vi "Engine_Build.vi"(8 "ErrIn":errorcluster, 9 "Programmatic?":bool, 10 "New item":T1, 11 "IB_MSI.lvclass":refnum<class "IB_MSI.lvclass">) -> (0 "ErrOut":errorcluster, 1 "warning":string, 2 "Canceled?":bool)   [LabVIEW 2020, in "IB_MSI.lvclass"]
uses:
  <vilib>/AppBuilder/IB_Classes/MSI/IB_MSI.lvclass
  AppLibs/distkit/MDF/NI_MDF.lvlib
  <resource>/Framework/Providers/Builds/Installer/CDK_GLOBAL_STRINGS.vi
  AppLibs/distkit/MDF/NIMdf.llb/MDFMIResourceStringID.ctl
  <vilib>/AppBuilder/IB_Classes/Installer/Installer.lvclass
  AppLibs/distkit/MDF/NIMdf.llb/MDFCommonOptions.ctl
  e:/builds/penguin/labview/branches/2020/dev/dist/vi.lib/AppBuilder/IB_Classes/Installer/Installer.lvclass
  e:/builds/penguin/labview/branches/2020/dev/dist/vi.lib/AppBuilder/IB_Classes/MSI/IB_MSI.lvclass
  <resource>/Framework/Providers/API/mxLvBuildNewItem.ctl
panel:
  out "#Vol":u32
  out "VolumeLabel":string
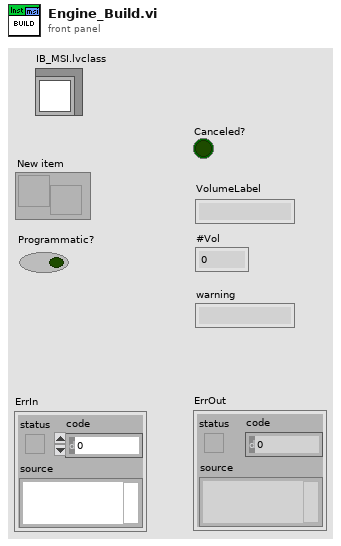
[diagram p1: front panel]
types:
  T1 = typedef "mxLvBuildNewItem.ctl" = refnum<user-event>
  T2 = cluster{"last known path":path, "Index":i32, "DistTitle":string}[]
  T3 = typedef "NI_MDF.lvlib/MDFMIResourceStringID.ctl" = i32
  T4 = typedef "IB_Installer.ctl" = cluster{"Destination":refnum<class "IB_Destination.lvclass">[], "Source":refnum<class "IB_Source.lvclass">[], "buildObject":T5, "defaultDir":string, "platform":string, "author":string, "productName":string, "buildSpecName":string, "hide":bool, "requireLVDevSys":bool, "autoIncrement":bool, "includeError":bool, "readmeID":string, "buildLocation":path, "readmePath":path, "mediaSize":u16, "language":T6, "productVersion":T7, "preview":bool, "programmatic":bool, "progressBarEvents":T8, "userLog_Path":path, "shortcutAddresses":T10[], "EXE_Install Address":string, "EXE_Uninstall Address":string, "additional NIPaths":refnum<class "Dest_NI_NIPath.lvclass">[], "web service itemIDs":string[], "installerName":string}
  T5 = typedef "ItemRef.ctl" = u64
  T6 = typedef "CDK_sTypeDef_Languages.ctl" = u16
  T7 = typedef "CDK_sTypeDef_ProductVersion.ctl" = cluster{"Major":u8, "Minor":u8, "Update":u16}
  T8 = typedef "provcom_ProgressBar_Events.ctl" = cluster{"newJob":refnum<user-event>, "newItem":refnum<user-event>, "errorMsg":T9, "cancel":refnum<user-event>}
  T9 = typedef "mxLvBuildError.ctl" = refnum<user-event>
  T10 = typedef "CDK_sTypeDef_ShortcutAddress.ctl" = cluster{"file":string, "shortcut":string}
  T11 = typedef "IB_MSI.ctl" = cluster{"upgradeCode":string, "distID":string, "windowMessage":string, "windowTitle":string, "arpPhone":string, "arpContact":string, "arpURL":string, "arpCompany":string, "licenseID":string, "licensePath":path, "welcomeImageID":string, "welcomeImagePath":path, "bannerImageID":string, "bannerImagePath":path, "osCheck":i32, "msiFileName":string, "cabFileName":string, "hwOption":T12, "hwPath":path, "regGroup":refnum<class "IB_RegGroup.lvclass">[], "regDest":refnum<class "IB_RegDest.lvclass">[], "selectedDists":refnum<class "IB_DistPart.lvclass">[], "installedDists":refnum<class "IB_DistPart.lvclass">[], "postInstallSteps":refnum<class "IB_Post_Install_Step.lvclass">[], "preUninstallSteps":refnum<class "IB_Post_Install_Step.lvclass">[], "winsec.certificate":string, "winsec.timestamp":string, "winsec.description":string, "autoselect drivers":bool, "hide non-runtimes":bool}
  T12 = typedef "CDK_sTypeDef_HWImportOption.ctl" = enum16{"<none>", "Merge", "Replace", "Dialog"}
  T13 = typedef "NI_MDF.lvlib/MDFCommonOptions.ctl" = i32
  T14 = cluster{"last known path":path, i32, "distribution name":string}
  T15 = cluster{"last known path":path, "Index":i32, "distribution name":string}[]
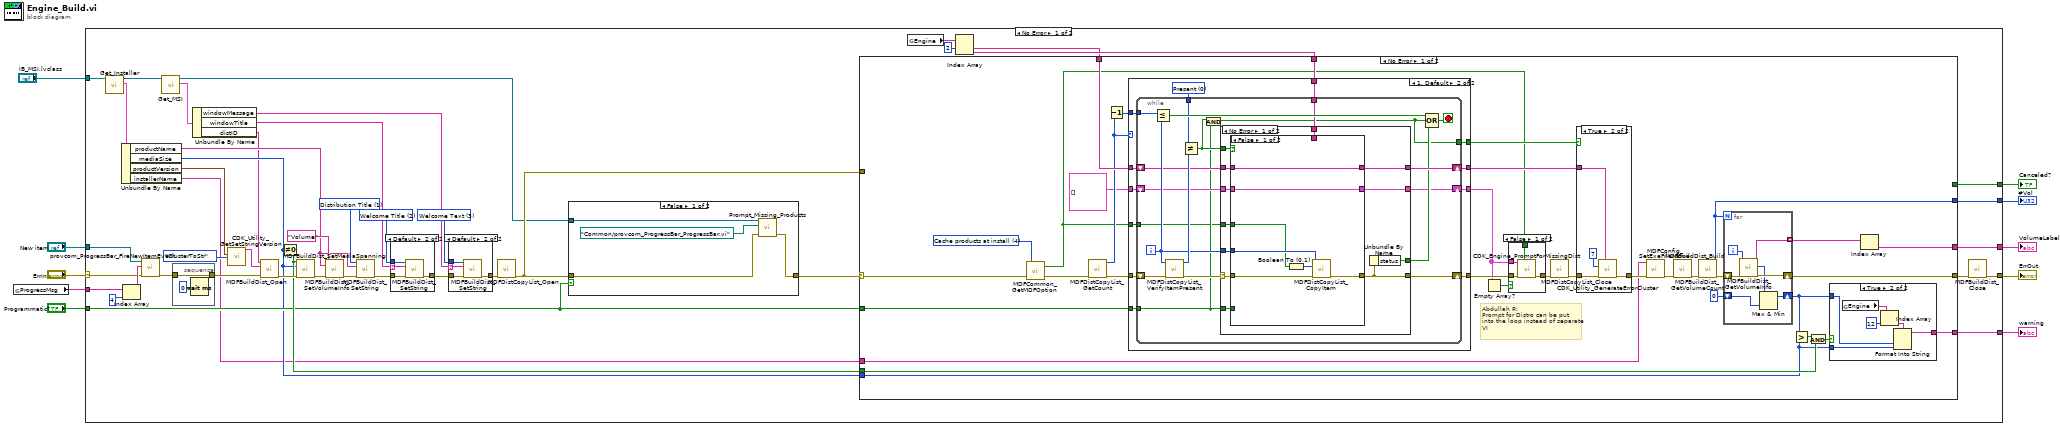
[diagram p0: block diagram]
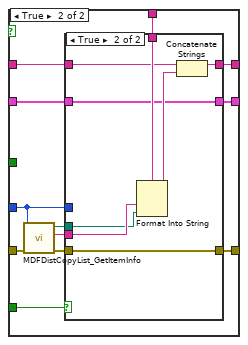
[diagram p5: hidden frame]
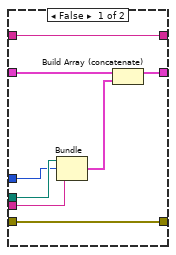
[diagram p6: hidden frame]
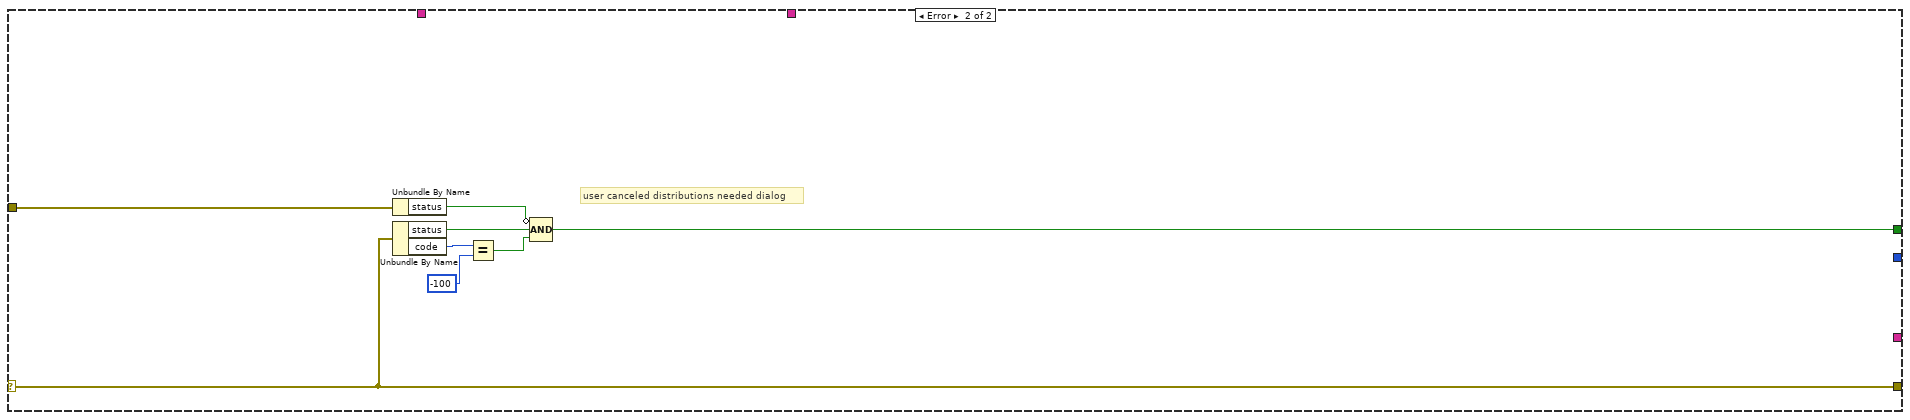
[diagram p9: hidden frame]
diagram:
  n1 = global read "CDK_GLOBAL_STRINGS.vi" "ProgressMsg"() -> (w5:string[])
  n2 = case shown="No Error" "ErrIn" {
    selector: "ErrIn" -> [w51 w219]
    tunnel: [w28 w219] -> w10
    tunnel: "New item" -> [w55 _]
    tunnel: [w36 _] -> w7
    tunnel: [w37 _] -> w6
    tunnel: w5 -> [w50 _]
    tunnel: "Programmatic?" -> [w32 _]
    tunnel: [w34 _] -> w3
    tunnel: [w30 _] -> w2
    tunnel: "IB_MSI.lvclass" -> [w23 _]
    frame No Error {
      w38 = T3 3 items=["Distribution Title"=1, "Welcome Title"=2, "Welcome Text"=3, "Single Directory Text 1"=4, "Single Directory Edit Label 1"=8, "Single Directory Edit Label 2"=9, "Single Directory Edit Label 3"=10, "Single Directory Edit Label 4"=11, "Single Directory Edit Label 5"=12, "Single Directory Edit Label 6"=13] ("MI ResourceString ID")
      w39 = T3 2 items=["Distribution Title"=1, "Welcome Title"=2, "Welcome Text"=3, "Single Directory Text 1"=4, "Single Directory Edit Label 1"=8, "Single Directory Edit Label 2"=9, "Single Directory Edit Label 3"=10, "Single Directory Edit Label 4"=11, "Single Directory Edit Label 5"=12, "Single Directory Edit Label 6"=13] ("MI ResourceString ID")
      w44 = T3 1 items=["Distribution Title"=1, "Welcome Title"=2, "Welcome Text"=3, "Single Directory Text 1"=4, "Single Directory Edit Label 1"=8, "Single Directory Edit Label 2"=9, "Single Directory Edit Label 3"=10, "Single Directory Edit Label 4"=11, "Single Directory Edit Label 5"=12, "Single Directory Edit Label 6"=13] ("MI ResourceString ID")
      n3 = call <vilib>:"Get_Installer.vi"("Installer in"=w23) -> ("data"=w22:T4, "Installer out"=w14:refnum<class "IB_MSI.lvclass">)  [unwired: 1 in, 8 out]
      n4 = Unbundle By Name(w22) -> ("productName"=w18:string, "mediaSize"=w17:u16, "productVersion"=w16:T7, "installerName"=w11:string)
      n5 = Index Array(array=w50, index=4) -> (element=w54:string)
      n6 = call <resource>:"provcom_ProgressBar_FireNewItemEvent.vi"("error in (no error)"=w51, "Label"=w54, "NewItem"=w55) -> ("error out"=w48:errorcluster)  [unwired: 8 out]
      n7 = call <vilib>:"Get_MSI.vi"("IB_MSI in"=w14) -> ("data"=w21:T11, "IB_MSI out"=w13:refnum<class "IB_MSI.lvclass">)  [unwired: 1 in, 8 out]
      n8 = stacked-sequence {
        tunnel: w48 -> [w217]
        tunnel: [w217] -> w47
        frame #0 {
          n9 = Wait (ms)(milliseconds to wait=u32 0) -> ()  [unwired: 1 out]
        }
      }
      n10 = Unbundle By Name(w21) -> ("windowMessage"=w20:string, "windowTitle"=w19:string, "distID"=w15:string)
      n11 = call <resource>:"CDK_Utility_GetSetStringVersion.vi"("Action"=enum16{"ClusterToStr", "StrToCluster"}."ClusterToStr", "ProductVersionIn"=w16) -> ("VersionStringOut"=w52:string)  [unwired: 2 in, 7 out]
      n12 = call "MDFBuildDist_Open.vi"("error in (no error)"=w47, "version (1.0.0)"=w52, "distribution Id (GUID)"=w15) -> ("error out"=w49:errorcluster)  [unwired: 8 out]
      n13 = Not Equal To 0?(x=w17) -> (x != 0?=w35:bool)
      n14 = call "MDFBuildDist_SetMediaSpanning.vi"("error in (no error)"=w49, "media size (MB)"=w17, "EnableMediaSpanning? (false)"=w35) -> ("error out"=w46:errorcluster)  [unwired: 8 out]
      n15 = call "MDFBuildDist_SetVolumeInfo.vi"("error in (no error)"=w46, "disk prompt"=w18, "volume label"="Volume") -> ("error out"=w43:errorcluster)  [unwired: 8 out]
      n16 = call "MDFBuildDist_SetString.vi"("error in (no error)"=w43, "String"=w18, "MI ResourceString ID"=w44) -> ("error out"=w42:errorcluster)  [unwired: 8 out]
      n17 = case shown="Default" w19 {
        selector: w19 -> [_ w215]
        tunnel: w42 -> [w212 w216]
        tunnel: [w212 w214] -> w41
        tunnel: w39 -> [_ w213]
        frame "" {
        }
        frame Default {
          n18 = call "MDFBuildDist_SetString.vi"("error in (no error)"=w216, "String"=w215, "MI ResourceString ID"=w213) -> ("error out"=w214:errorcluster)  [unwired: 8 out]
        }
      }
      n19 = case shown="Default" w20 {
        selector: w20 -> [_ w210]
        tunnel: w41 -> [w207 w211]
        tunnel: [w207 w209] -> w40
        tunnel: w38 -> [_ w208]
        frame "" {
        }
        frame Default {
          n20 = call "MDFBuildDist_SetString.vi"("error in (no error)"=w211, "String"=w210, "MI ResourceString ID"=w208) -> ("error out"=w209:errorcluster)  [unwired: 8 out]
        }
      }
      n21 = call "MDFDistCopyList_Open.vi"("error in (no error)"=w40) -> ("error out"=w31:errorcluster)  [unwired: 10 out]
      n22 = case shown="False" w32 {
        tunnel: w31 -> [w203 w206]
        tunnel: [w202 w206] -> w12
        tunnel: w13 -> [w205 _]
        frame False {
          n23 = call <vilib>:"Prompt_Missing_Products.vi"("error in"=w203, "parent VI path"=path "Common/provcom_ProgressBar_ProgressBar.vi" ("vi path"), "Class"=w205) -> ("error out"=w202:errorcluster)  [unwired: 1 in, 7 out]
        }
        frame True {
          # "bpreis: let build fail\nif deployable parts\nare missing during\nprogrammatic build"
        }
      }
      n24 = global read "CDK_GLOBAL_STRINGS.vi" "Engine"() -> (w26:string[])
      n25 = Index Array(array=w26, index #1=2 ("index")) -> (element #1=w24:string, element #2=w25:string)  [unwired: 1 in]
      n26 = case shown="No Error" w12 {
        selector: w12 -> [w62 w200]
        tunnel: [w61 w200] -> w29
        tunnel: w25 -> [w84 _]
        tunnel: w24 -> [w82 _]
        tunnel: [w72 _] -> w37
        tunnel: [w71 _] -> w36
        tunnel: w35 -> [w68 _]
        tunnel: w17 -> [w65 _]
        tunnel: [w64 _] -> w34
        tunnel: w32 -> [w63 _]
        tunnel: w31 -> [_ w201]
        tunnel: [_ w194] -> w30
        tunnel: w11 -> [w56 _]
        frame No Error {
          w59 = T13 4 items=["Include patch targets with patches"=1, "Cache products at disk prompt"=2, "Cache products at install"=4] ("option to get")
          # "Abdullah R:\nPrompt for Distro can be put\ninto the loop instead of separate\nVI"
          n27 = call "MDFCommon_GetMDFOption.vi"("option to get"=w59) -> ("option value"=w60:bool)  [unwired: 1 in, 1 out]
          n28 = call "MDFDistCopyList_GetCount.vi"("error in (no error)"=w62) -> ("error out"=w88:errorcluster, "count"=w81:i32)  [unwired: 9 out]
          n29 = Decrement(x=w81) -> (x-1=w85:i32)
          n30 = case shown="1, Default" w81 {
            tunnel: w88 -> [w107 w119]
            tunnel: w85 -> [_ w118]
            tunnel: w84 -> [_ w117]
            tunnel: [_ w116] -> w74
            tunnel: [_ w115] -> w80
            tunnel: [w107 w114] -> w78
            tunnel: w82 -> [_ w113]
            tunnel: w63 -> [_ w112]
            tunnel: T2 [] -> [_ w110]
            tunnel: [_ w109] -> w76
            tunnel: w60 -> [_ w108]
            frame 0 {
            }
            frame 1, Default {
              w111 = 0 items=["Present", "Not a Distribution", "Removable media not present", "Network location not accessible", "Path not found", "Incorrect Distribution"] ("reason missing")
              n31 = while {
                shift-right: [w132] -> w114
                shift-left: w119 -> [w138]
                tunnel: w118 -> [w137]
                tunnel: w111 -> [w133]
                tunnel: w117 -> [w129]
                shift-right: [w127] -> w115
                shift-left: w113 -> [w128]
                tunnel: [w121] -> w116
                tunnel: w112 -> [w122]
                shift-right: [w124] -> w109
                shift-left: w110 -> [w125]
                tunnel: w108 -> [w120]
                i -> [w130]
                stop <- w134 stop-if-true
                n32 = Less Or Equal?(x=w137, y=w130) -> (x <= y?=w135:bool)
                n33 = call "MDFDistCopyList_VerifyItemPresent.vi"("error in (no error)"=w138, "index"=w130) -> ("error out"=w131:errorcluster, "reason missing"=w136:i32)  [unwired: 8 out]
                n34 = Not Equal?(x=w133, y=w136) -> (x != y?=w123:bool)
                n35 = And(x=w123, y=w122) -> (x .and. y?=w121:bool)
                n36 = case shown="No Error" w131 {
                  selector: w131 -> [w149 w188]
                  tunnel: [w144 w188] -> w132
                  tunnel: w123 -> [w150 _]
                  tunnel: w130 -> [w148 _]
                  tunnel: w129 -> [w147 _]
                  tunnel: w128 -> [w146 w187]
                  tunnel: [w145 w187] -> w127
                  tunnel: [w143 _] -> w126
                  tunnel: w122 -> [w142 _]
                  tunnel: w125 -> [w141 w186]
                  tunnel: [w140 w186] -> w124
                  tunnel: w120 -> [w139 _]
                  frame No Error {
                    n37 = case shown="False" w150 {
                      tunnel: w149 -> [w157 w164]
                      tunnel: [w156 w169] -> w144
                      tunnel: w148 -> [w155 w160]
                      tunnel: w147 -> [_ w168]
                      tunnel: w146 -> [w154 w167]
                      tunnel: [w154 w166] -> w145
                      tunnel: w142 -> [_ w165]
                      tunnel: w141 -> [w153 w159]
                      tunnel: [w153 w158] -> w140
                      tunnel: w139 -> [w151 _]
                      frame False {
                        n38 = Boolean To (0,1)(Boolean=w151) -> (0, 1=w152:i16)
                        n39 = call "MDFDistCopyList_CopyItem.vi"("error in (no error)"=w157, "cache products"=w152, "index"=w155) -> ("error out"=w156:errorcluster)  [unwired: 1 in, 7 out]
                      }
                      frame True {
                        n40 = call "MDFDistCopyList_GetItemInfo.vi"("error in (no error)"=w164, "index"=w160) -> ("error out"=w161:errorcluster, "distribution name"=w163:string, "last known path"=w162:path)  [unwired: 7 out]
                        n41 = case shown="True" w165 {
                          tunnel: [w176 w179] -> w169
                          tunnel: w168 -> [_ w185]
                          tunnel: w167 -> [w177 w184]
                          tunnel: [w177 w182] -> w166
                          tunnel: w163 -> [w172 w181]
                          tunnel: w162 -> [w175 w180]
                          tunnel: w161 -> [w176 w179]
                          tunnel: w160 -> [w171 _]
                          tunnel: w159 -> [w174 w178]
                          tunnel: [w173 w178] -> w158
                          frame False {
                            n42 = Bundle("last known path"=w175, w171, "distribution name"=w172) -> (w170:T14)  [unwired: 1 out]
                            n43 = Build Array (concatenate)(w174, w170) -> (w173:T15)
                          }
                          frame True {
                            n44 = Format Into String(format string=w185, w181, w180) -> (resulting string=w183:string)  [unwired: 2 in, 1 out]
                            n45 = Concatenate Strings(w184, w183) -> (w182:string)
                          }
                        }
                      }
                    }
                    n46 = Unbundle By Name(w144) -> ("status"=w143:bool)
                  }
                  frame Error {
                  }
                }
                n47 = Compound Arithmetic op=OR(w135, w121, w126) -> (w134:bool)
              }
            }
          }
          n48 = Empty Array?(array=w76) -> (empty?=w75:bool)
          n49 = case shown="False" w75 {
            tunnel: w78 -> [w105 w106]
            tunnel: [w104 w106] -> w77
            tunnel: w76 -> [w103 _]
            tunnel: w60 -> [w102 _]
            frame False {
              n50 = call <resource>:"CDK_Engine_PromptForMissingDist.vi"("CacheDistros"=w102, "ErrIn"=w105, "MissingLocs"=w103) -> ("ErrOut"=w104:errorcluster)  [unwired: 8 out]
            }
            frame True {
            }
          }
          n51 = call "MDFDistCopyList_Close.vi"("error in (no error)"=w77) -> ("error out"=w83:errorcluster)  [unwired: 10 out]
          n52 = case shown="True" w74 {
            tunnel: w83 -> [w189 w193]
            tunnel: w80 -> [_ w191]
            tunnel: [w189 w192] -> w58
            frame False {
            }
            frame True {
              n53 = call <resource>:"CDK_Utility_GenerateErrorCluster.vi"("Additional Info"=w191, "ErrIn"=w193, "code"=7) -> ("ErrOut"=w192:errorcluster)  [unwired: 1 in, 7 out]
            }
          }
          n54 = call "MDFConfig_SetExeFileName.vi"("error in (no error)"=w58, "exe filename"=w56) -> ("error out"=w57:errorcluster)  [unwired: 9 in]
          n55 = call "MDFBuildDist_Build.vi"("error in (no error)"=w57) -> ("error out"=w87:errorcluster)  [unwired: 10 out]
          n56 = call "MDFBuildDist_GetVolumeCount.vi"("error in (no error)"=w87) -> ("error out"=w86:errorcluster, "number of volumes created"=w72:i32)  [unwired: 9 out]
          n57 = for {
            N: w72 -> [_]
            tunnel: [w99] -> w70 mode=indexing
            shift-right: [w101] -> w61
            shift-left: w86 -> [w100]
            shift-right: [w97] -> w66
            shift-left: 0 -> [w96]
            i -> [w95]
            n58 = call "MDFBuildDist_GetVolumeInfo.vi"("error in (no error)"=w100, "index"=w95) -> ("error out"=w101:errorcluster, "final media cost"=w98:u32, "volume label"=w99:string)  [unwired: 7 out]
            n59 = Max & Min(x=w98, y=w96) -> (max(x,y)=w97:u32)  [unwired: 1 out]
          }
          n60 = Greater?(x=w66, y=w65) -> (0:w69:bool)
          n61 = And(x=w69, y=w68) -> (x .and. y?=w67:bool)
          n62 = case shown="True" w67 {
            tunnel: w66 -> [_ w91]
            tunnel: w65 -> [_ w90]
            tunnel: [_ w89] -> w64
            frame False {
            }
            frame True {
              n63 = global read "CDK_GLOBAL_STRINGS.vi" "Engine"() -> (w94:string[])
              n64 = Index Array(array=w94, index=12) -> (element=w92:string)
              n65 = Format Into String(format string=w92, w91, w90) -> (resulting string=w89:string)  [unwired: 2 in, 1 out]
            }
          }
          n66 = Index Array(array=w70) -> (element=w71:string)  [unwired: 1 in]
        }
        frame Error {
          # "user canceled distributions needed dialog"
          n67 = Unbundle By Name(w201) -> ("status"=w195:bool)
          n68 = Unbundle By Name(w200) -> ("status"=w196:bool, "code"=w199:i32)
          n69 = Equal?(x=w199, y=-100) -> (x = y?=w197:bool)
          n70 = Compound Arithmetic op=AND(invert w195, w196, w197) -> (w194:bool)
        }
      }
      n71 = call "MDFBuildDist_Close.vi"("error in (no error)"=w29) -> ("error out"=w28:errorcluster)  [unwired: 10 out]
    }
    frame Error {
    }
  }
  "ErrOut" <- w10
  "VolumeLabel" <- w7
  "#Vol" <- w6
  "warning" <- w3
  "Canceled?" <- w2
